vi "Test serialization.vi"() -> ()   [LabVIEW 2014]
uses:
  <vilib>/NI/AQ Character Lineator/JSON Serializer/JSON Serializer.lvclass
  <vilib>/NI/AQ Character Lineator/Formatter/Path Embedding.ctl
  <vilib>/NI/AQ Character Lineator/Serialization Common/Serial Version.ctl
  Reusable/CRDS/Data/Cell/CRDS Cell Data.lvclass
  <vilib>/NI/AQ Character Lineator/JSON Serializer/JSON Serializer.lvclass/JSON Serializer.ctl
  <vilib>/NI/AQ Character Lineator/Formatter/Formatter.lvclass/Formatter.ctl
  <vilib>/NI/AQ Character Lineator/Formatter/Formatter.lvclass
  <vilib>/NI/AQ Character Lineator/Serializer/Serializer.lvclass
  <vilib>/NI/AQ Character Lineator/Serialization Common/Serialization Common.lvlib
panel:
  out "Numeric":u32
  out "String":string
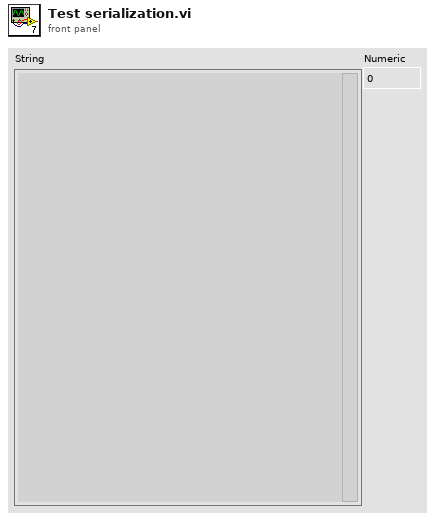
[diagram p1: front panel]
types:
  T1 = typedef "Serialization Common.lvlib/Serial Version.ctl" = cluster{"Major":u16, "Minor":u16, "Fix":u16, "Build":u16}
  T2 = typedef "Formatter.lvclass/Path Embedding.ctl" = enum16{"No paths embedded", "One path with each object", "All paths with each top object"}
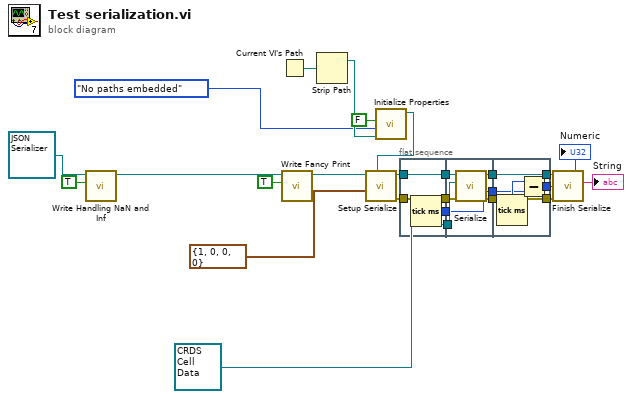
[diagram p0: block diagram]
diagram:
  n1 = call <vilib>:"Write Handling NaN and Inf.vi"("Allow encoding NaN and Infinity?"=TRUE, "JSON Serializer in"=refnum<class "JSON Serializer.lvclass"> refnum ("TestSerializer.lvclass")) -> ("JSON Serializer out"=w23:refnum<class "JSON Serializer.lvclass">)  [unwired: 9 in]
  n2 = Current VI's Path() -> (path=w21:path)
  n3 = call <vilib>:"Write Fancy Print.vi"("Fancy Print"=TRUE, "JSON Serializer in"=w23) -> ("JSON Serializer out"=w22:refnum<class "JSON Serializer.lvclass">)  [unwired: 9 in]
  n4 = Strip Path(path=w21) -> (stripped path=w20:path)  [unwired: 1 out]
  n5 = call <vilib>:"Initialize Properties.vi"("Absolute Path For Dynamic Loading"=w20, "Dynamic Path Behavior"=Path_Embedding."No paths embedded", "Include Default Values? (T)"=FALSE) -> ("Formatter out"=w19:refnum<class "Formatter.lvclass">)  [unwired: 8 in]
  n6 = call <vilib>:"Setup Serialize.vi"("Formatter (defaults)"=w19, "Serial Version"=T1 {"Major"=1, "Minor"=0, "Fix"=0, "Build"=0}, "Serializer in"=w22) -> ("error out"=w10:errorcluster, "Serializer out"=w17:refnum<class "JSON Serializer.lvclass">)  [unwired: 7 in]
  n7 = flat-sequence {
    tunnel: w10 -> [w26]
    tunnel: w17 -> [w27]
    tunnel: [w27] -> w5
    tunnel: [w26] -> w4
    tunnel: [w25] -> w3
    tunnel: refnum<class "CRDS Cell Data.lvclass"> refnum ("CRDS Cell") -> [w29]
    tunnel: [w32] -> w7
    tunnel: [w31] -> w6
    tunnel: w5 -> [w33]
    tunnel: w4 -> [w30]
    tunnel: w3 -> [w28]
    tunnel: [w28] -> w2
    tunnel: [w37] -> w11
    tunnel: [w38] -> w12
    tunnel: w7 -> [w38]
    tunnel: w6 -> [w37]
    tunnel: w2 -> [w35]
    tunnel: [w34] -> w1
    frame #0 {
      n8 = Tick Count (ms)() -> (millisecond timer value=w25:u32)
    }
    frame #1 {
      n9 = call-dynamic "Serialize.vi"("error in (no error)"=w30, "Serializable"=w29, "JSON Serializer in"=w33) -> ("error out"=w31:errorcluster, "JSON Serializer out"=w32:refnum<class "JSON Serializer.lvclass">)  [unwired: 7 in]
    }
    frame #2 {
      n10 = Tick Count (ms)() -> (millisecond timer value=w36:u32)
      n11 = Subtract(x=w36, y=w35) -> (x-y=w34:u32)
    }
  }
  n12 = call <vilib>:"Finish Serialize.vi"("error in (no error)"=w11, "Serializer in"=w12) -> ("String"=→"String":string)  [unwired: 6 in, 3 out]
  "Numeric" <- w1
